vi "SigmaCutterFilter.vi"(11 "Spiky\n   Vmag         U             V             W          Cone":dbl[][](array[numeric]) caption="SpikyData") -> (3 "Cleaned\n   Vmag          U               V              W        Cone":dbl[][](array[numeric]) caption="De-spikedData")   [LabVIEW 2016]
panel:
  in  "+/-Nsigma":dbl=3.0
  out "Stats-postfilter":dbl[][](array[numeric])
  out "Stats-prefilter":dbl[][](array[numeric])
  # "Mean"
  # "Var"
  # "Skew"
  # "Kurt"
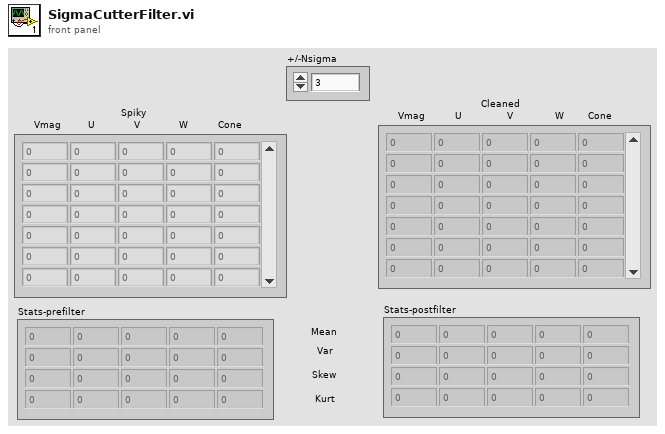
[diagram p1: front panel]
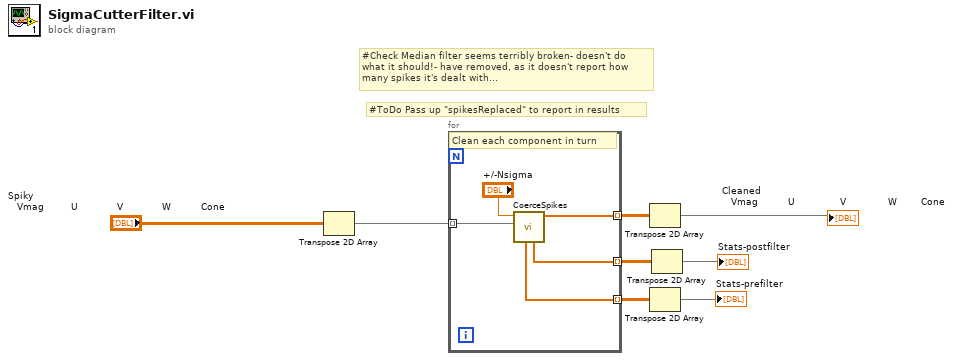
[diagram p0: block diagram]
diagram:
  # "#ToDo Pass up \"spikesReplaced\" to report in results"
  # "#Check Median filter seems terribly broken- doesn't do what it should!- have removed, as it doesn't report how many spikes it's dealt with..."
  n1 = Transpose 2D Array(2D array="Spiky\n   Vmag         U             V             W          Cone") -> (transposed array=w5:dbl[][])
  n2 = for {
    tunnel: w5 -> [w12] mode=indexing
    tunnel: [w10] -> w6 mode=indexing
    tunnel: [w11] -> w4 mode=indexing
    tunnel: [w9] -> w3 mode=indexing
    # "Clean each component in turn"
    n3 = call "CoerceSpikes.vi"("spikyData"=w12, "+/-Nsigma"="+/-Nsigma") -> ("deSpikedData"=w10:dbl[], "CleanStats"=w9:dbl[], "SpikyStats"=w11:dbl[])  [unwired: 6 in, 1 out]
  }
  n4 = Transpose 2D Array(2D array=w6) -> (transposed array=→"Cleaned\n   Vmag          U               V              W        Cone":dbl[][])
  n5 = Transpose 2D Array(2D array=w4) -> (transposed array=→"Stats-prefilter":dbl[][])
  n6 = Transpose 2D Array(2D array=w3) -> (transposed array=→"Stats-postfilter":dbl[][])
